vi "Initialize Work.vi"(8 "error in (no error)":errorcluster, 9 "Update period":dbl, 10 "Reply to":refnum<class "Result Reply Msg.lvclass">, 11 "Measure Controller in":refnum<class "Process Controller.lvclass">) -> (0 "error out":errorcluster, 3 "Measure Controller out":refnum<class "Process Controller.lvclass">)   [LabVIEW 2016, in "Process Controller.lvclass"]
uses:
  Process Controller.lvclass
  C:/github/LabActor/Worker/Worker.lvclass
  Template Module Messages/Result Reply Msg/Result Reply Msg.lvclass
  Process Controller Messages/Init Response Msg/Init Response Msg.lvclass
  C:/github/LabActor/Template Module Messages/Result Reply Msg/Result Reply Msg.lvclass
  Worker/Worker.lvclass/Worker.ctl
  NHMFL_Core/Libraries/Instruments/Results/Acquired Result/Acquired Result.lvclass
  Worker Messages/Initialize Work Msg/Initialize Work Msg.lvclass/Initialize Work Msg.ctl
  <vilib>/ActorFramework/Message Enqueuer/Message Enqueuer.lvclass/Message Enqueuer.ctl
  Process Controller.lvclass/Process Controller.ctl
  Worker/Write Pause requested.vi
  Worker/Write Paused.vi
  <vilib>/ActorFramework/Message Enqueuer/Enqueue.vi
  Worker Messages/Initialize Work Msg/Initialize Work Msg.lvclass
  C:/Program Files/National Instruments/LabVIEW 2016/vi.lib/ActorFramework/Message/Message.lvclass
  <vilib>/ActorFramework/Message Priority Queue/Priority Enqueue.vi
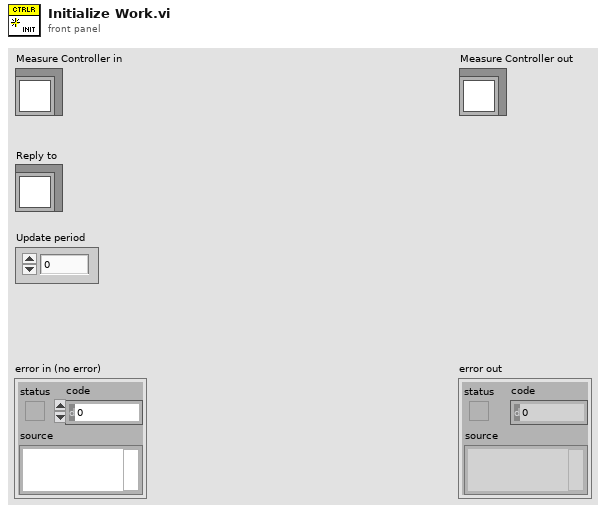
[diagram p1: front panel]
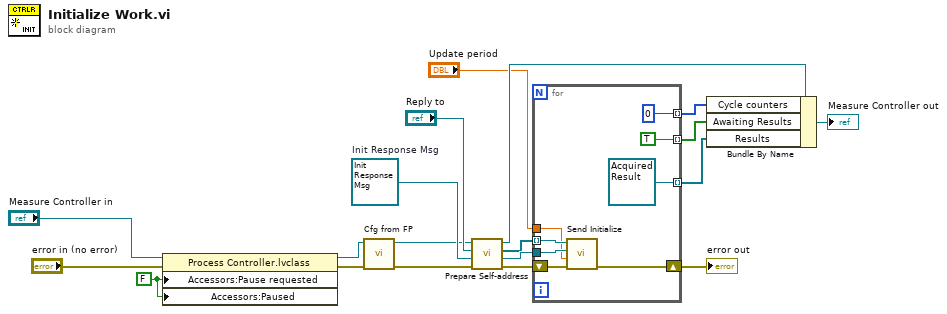
[diagram p0: block diagram]
diagram:
  w1 = FALSE ("Pause requested")
  w10 = refnum<class "Init Response Msg.lvclass"> refnum  # Init Response Msg
  n1 = property class="Process Controller.lvclass"(reference="Measure Controller in", error in="error in (no error)", "Accessors:Pause requested"=w1, "Accessors:Paused"=w1) -> (reference out=w2:refnum<class "Process Controller.lvclass">, error out=w4:errorcluster)
  n2 = call-dynamic "Cfg from FP.vi"("error in (no error)"=w4, "Measure Object in"=w2) -> ("error out"=w8:errorcluster, "Measure Object out"=w7:refnum<class "Process Controller.lvclass">)  [unwired: 8 in]
  n3 = call-dynamic "Prepare Self-address.vi"("error in (no error)"=w8, "Reply to me"=w10, "Reply to"="Reply to", "Process Controller in"=w7) -> ("error out"=w12:errorcluster, "Reply to me"=w14:refnum<class "Result Reply Msg.lvclass">, "Active measurements enqueuers"=w13:refnum<class "Message Enqueuer.lvclass">[], "Process Controller out"=w11:refnum<class "Process Controller.lvclass">)  [unwired: 4 in]
  n4 = for {
    tunnel: w13 -> [w23] mode=indexing
    shift-right: [w27] -> w16
    shift-left: w12 -> [w22]
    tunnel: [TRUE] -> w19 mode=indexing
    tunnel: [refnum<class "Acquired Result.lvclass"> refnum ("Placeholder Result")] -> w18 mode=indexing
    tunnel: w14 -> [w24]
    tunnel: "Update period" -> [w21]
    tunnel: [0] -> w5 mode=indexing
    n5 = call "Send Initialize.vi"("error in (no error)"=w22, "Cycle period"=w21, "Reply to"=w24, "Message Enqueuer"=w23) -> ("error out"=w27:errorcluster)  [unwired: 6 in, 1 out]
  }
  "error out" <- w16
  n6 = Bundle By Name(cluster=w11, "Cycle counters"=w5, "Awaiting Results"=w19, "Results"=w18) -> (→"Measure Controller out":refnum<class "Process Controller.lvclass">)
